vi "MH_SetInputChannels.vi"(10 "Channels new":T1[](array[typedef]) {"DeadTime" min=800 max=160000 step=1; "Edge" items=["falling", "rising"]; "Offset" min=-100000 max=100000 step=80; "Level" min=-1200 max=1200 step=1}, 11 "Channels old":T1[](array[typedef]) {"DeadTime" min=800 max=160000 step=1; "Edge" items=["falling", "rising"]; "Offset" min=-100000 max=100000 step=80; "Level" min=-1200 max=1200 step=1}) -> (2 "SetInpChan":T2[](array[typedef]), 3 "Channels":T1[](array[typedef]) {"DeadTime" min=800 max=160000 step=1; "Edge" items=["falling", "rising"]; "Offset" min=-100000 max=100000 step=80; "Level" min=-1200 max=1200 step=1})   [LabVIEW 2010]
uses:
  Types/MH_SetInpChanData.ctl
  Types/MH_SetInpChanCmds.ctl
  Types/MH_InputChannel.ctl
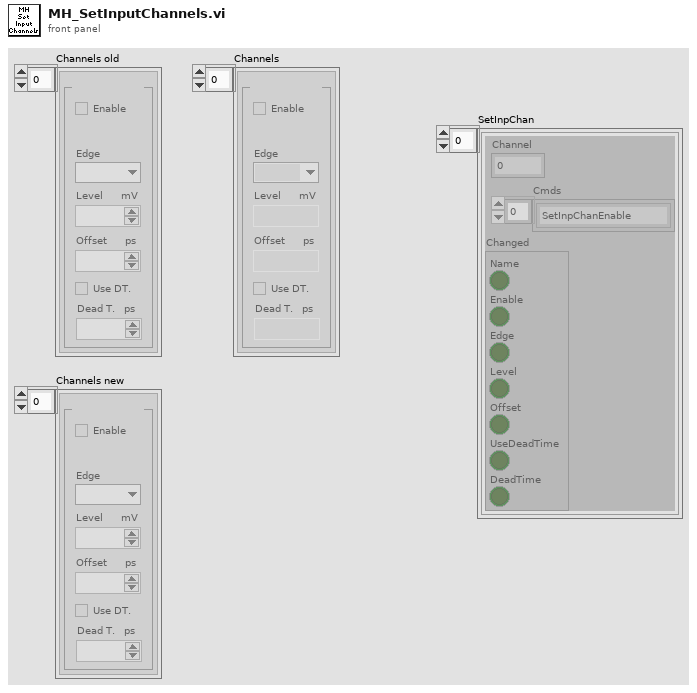
[diagram p1: front panel]
types:
  T1 = typedef "MH_InputChannel.ctl" = cluster{"Name":string, "Enable":bool, "Edge":i32, "Level":i32, "Offset":i32, "UseDeadTime":bool, "DeadTime":i32}
  T2 = typedef "MH_SetInpChanData.ctl" = cluster{"Channel":i32, "Cmds":T3[], "Changed":cluster{"Name":bool, "Enable":bool, "Edge":bool, "Level":bool, "Offset":bool, "UseDeadTime":bool, "DeadTime":bool}}
  T3 = typedef "MH_SetInpChanCmds.ctl" = enum16{"SetInpChanEnable", "SetInpChanOffset", "SetInpChanDeadTime", "SetInpChanTrg"}
  T4 = cluster{"Name":bool, "Enable":bool, "Edge":bool, "Level":bool, "Offset":bool, "UseDeadTime":bool, "DeadTime":bool}[]
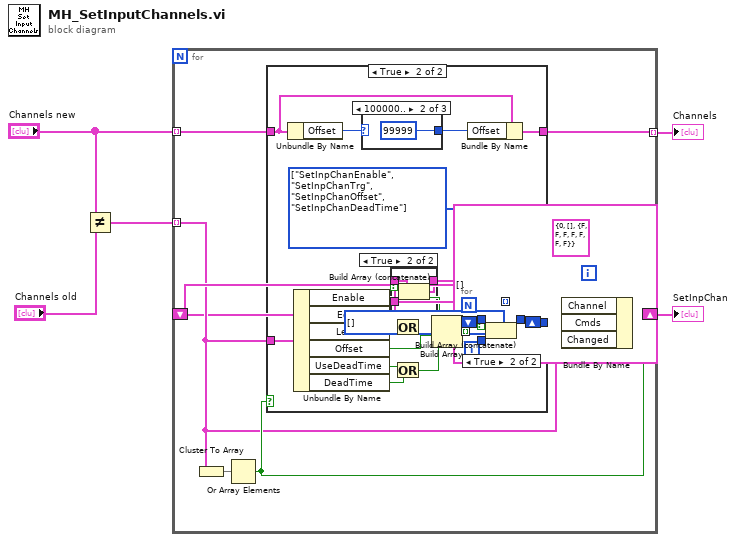
[diagram p0: block diagram]
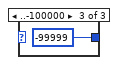
[diagram p5: hidden frame]
diagram:
  n1 = Not Equal?(x="Channels old", y="Channels new") -> (x != y?=w3:T4)
  n2 = for {
    tunnel: w3 -> [w9] mode=indexing
    tunnel: "Channels new" -> [w15] mode=indexing
    tunnel: [w14] -> w5 mode=indexing
    shift-right: [w7] -> w6
    shift-left: T2[] [] ("Array") -> [w8]
    i -> [w12]
    n3 = Cluster To Array(cluster=w9) -> (array=w17:bool[])
    n4 = Or Array Elements(Boolean array=w17) -> (logical OR=w16:bool)
    n5 = case shown="True" w16 {
      tunnel: w9 -> [_ w39]
      tunnel: [_ w29] -> w11
      tunnel: w15 -> [w22 w27]
      tunnel: [w22 w25] -> w14
      frame False {
      }
      frame True {
        w23 = T3[] [] items=["SetInpChanEnable", "SetInpChanOffset", "SetInpChanDeadTime", "SetInpChanTrg"] ("Array")
        w24 = T3[] [enum."SetInpChanEnable", enum."SetInpChanTrg", enum."SetInpChanOffset", enum."SetInpChanDeadTime"] items=["SetInpChanEnable", "SetInpChanOffset", "SetInpChanDeadTime", "SetInpChanTrg"]
        n6 = Unbundle By Name(w27) -> ("Offset"=w28:i32)
        n7 = Unbundle By Name(w39) -> ("Enable"=w34:bool, "Edge"=w36:bool, "Level"=w35:bool, "Offset"=w32:bool, "UseDeadTime"=w37:bool, "DeadTime"=w38:bool)
        n8 = case shown="100000.." w28 {
          selector: w28 -> [w40 _ _]
          tunnel: [w40 99999 ("SyncOffset") -99999 ("SyncOffset")] -> w26
          frame Default {
          }
          frame 100000.. {
          }
          frame ..-100000 {
          }
        }
        n9 = Or(x=w36, y=w35) -> (x .or. y?=w33:bool)
        n10 = Or(x=w37, y=w38) -> (x .or. y?=w31:bool)
        n11 = Build Array(w34, w33, w32, w31) -> (w30:bool[])
        n12 = for {
          tunnel: w30 -> [w45] mode=indexing
          tunnel: w24 -> [w46] mode=indexing
          shift-right: [w43] -> w29
          shift-left: w23 -> [w44]
          n13 = case shown="True" w45 {
            tunnel: w44 -> [w47 w49]
            tunnel: w46 -> [_ w48]
            tunnel: [w47 w50] -> w43
            frame False {
            }
            frame True {
              n14 = Build Array (concatenate)(w49, w48) -> (w50:T3[])
            }
          }
        }
        n15 = Bundle By Name(cluster=w27, "Offset"=w26) -> (w25:T1)
      }
    }
    n16 = Bundle By Name(cluster=T2 {"Channel"=0, "Cmds"=[], "Changed"={"Name"=FALSE, "Enable"=FALSE, "Edge"=FALSE, "Level"=FALSE, "Offset"=FALSE, "UseDeadTime"=FALSE, "DeadTime"=FALSE}}, "Channel"=w12, "Cmds"=w11, "Changed"=w9) -> (w10:T2)
    n17 = case shown="True" w16 {
      tunnel: w8 -> [w18 w20]
      tunnel: w10 -> [_ w19]
      tunnel: [w18 w21] -> w7
      frame False {
      }
      frame True {
        n18 = Build Array (concatenate)(w20, w19) -> (w21:T2[])
      }
    }
  }
  "SetInpChan" <- w6
  "Channels" <- w5
